vi "ChangeScale.vi"(11 "Probabilidade":dbl) -> (3 "changed probability":dbl)   [LabVIEW 2017]
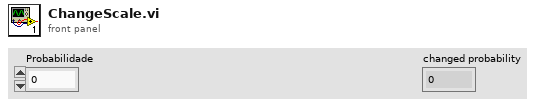
[diagram p1: front panel]
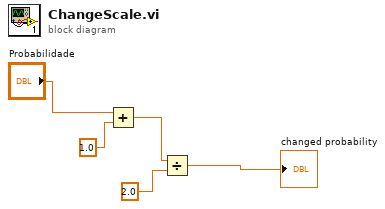
[diagram p0: block diagram]
diagram:
  n1 = Add(x="Probabilidade", y=1.0) -> (x+y=w3:dbl)
  n2 = Divide(x=w3, y=2.0) -> (x/y=→"changed probability":dbl)
